vi "Process_All_single.vi"(8 "error in (no error)":errorcluster, 11 "DebuggingTerminal":refnum<class "DebuggingTerminal.lvclass">) -> ()   [LabVIEW 2013, in "MQTT Base.lvlib"]
uses:
  MQTT Base.lvlib
  DebuggingTerminal.lvclass
  Packet Arrival -- cluster.ctl
  <vilib>/LabVIEW Open Source Project/MQTT Control Packets/Control Packets/ControlPacket/ControlPacket.lvclass
  DebuggingTerminal.lvclass/DebuggingTerminal.ctl
  <vilib>/LabVIEW Open Source Project/MQTT Control Packets/Control Packets/ControlPacket/ControlPacket.lvclass/ControlPacket.ctl
  <vilib>/LabVIEW Open Source Project/MQTT Control Packets/Control Packets/MQTT_311/MQTTVersion.lvclass
  <vilib>/LabVIEW Open Source Project/Advanced Structures/Circular Buffers/VariantBuffer/VariantBuffer.lvclass
  PacketFormatter/PacketFormatter.lvclass
panel:
  in  "auto-scroll":bool=TRUE
  out "Incoming":string
  # "MQTT Packets"
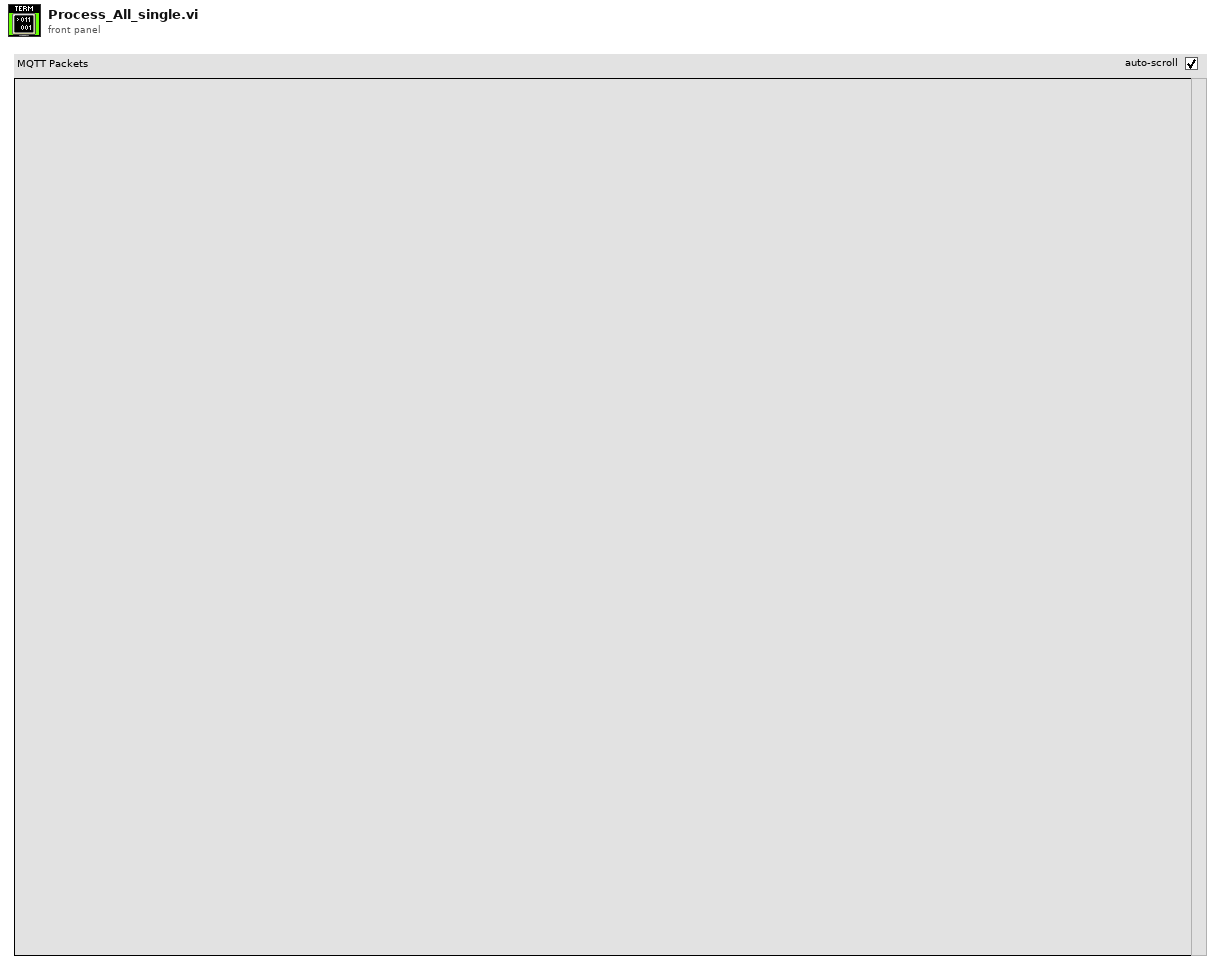
[diagram p1: front panel]
types:
  T1 = typedef "MQTT Base.lvlib/DebuggingTerminal.lvclass/Packet Arrival -- cluster.ctl" = cluster{"Timestamp":timestamp, "Packet":refnum<class "ControlPacket.lvclass">, "Session ID":i32, "outgoing":bool}
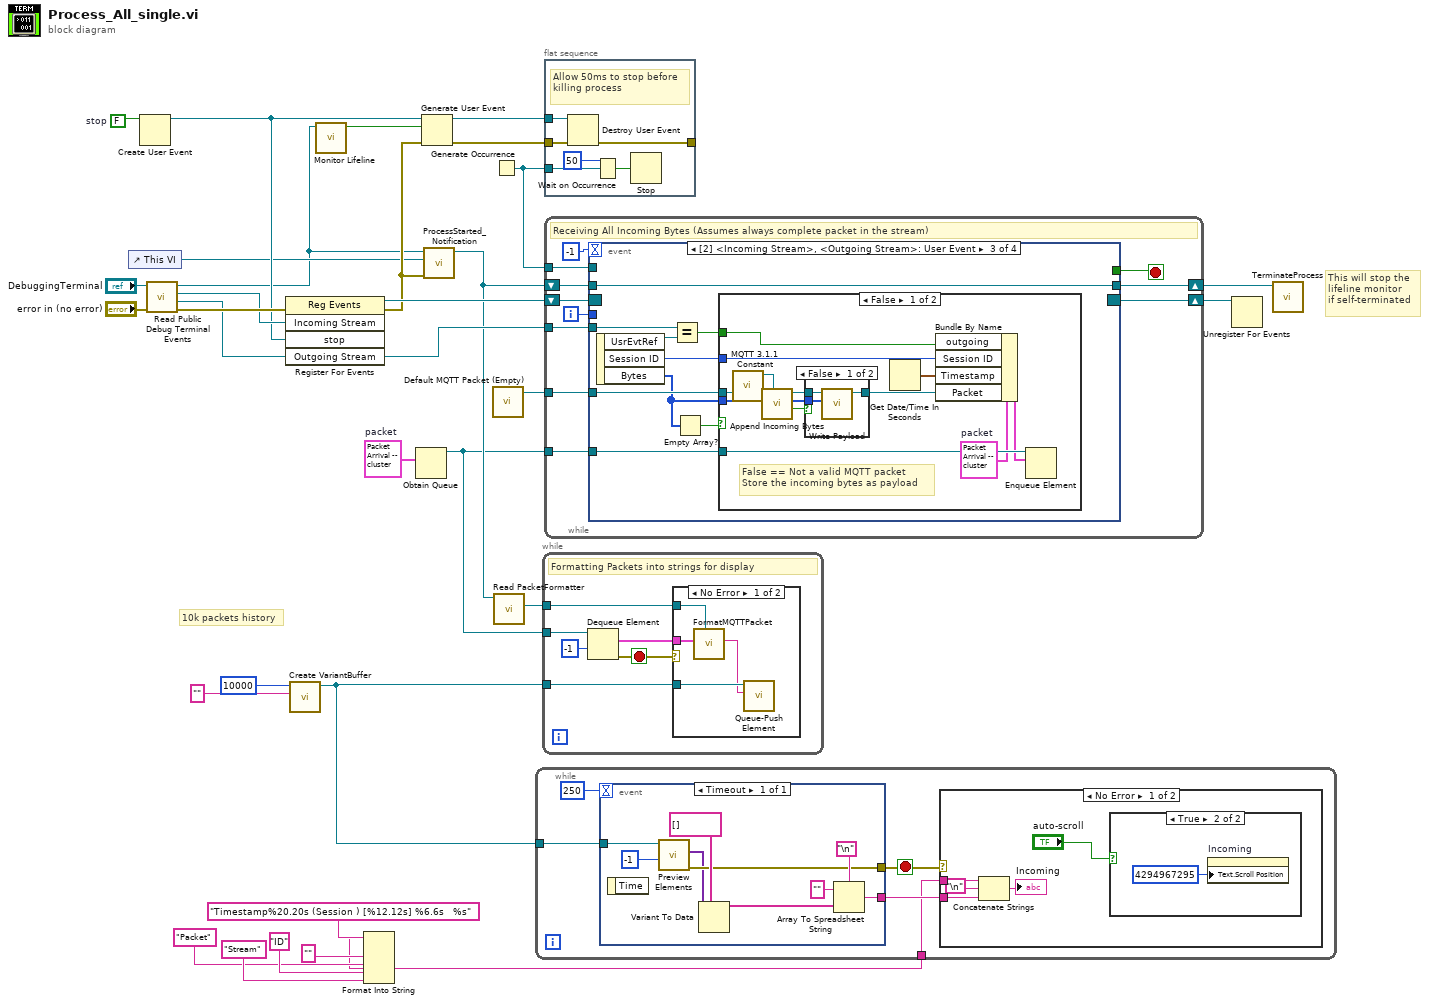
[diagram p0: block diagram]
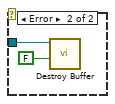
[diagram p2: hidden frame]
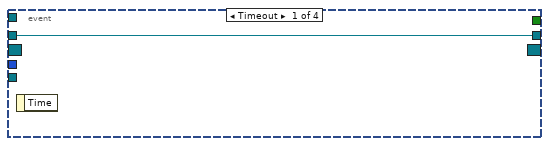
[diagram p5: hidden frame]
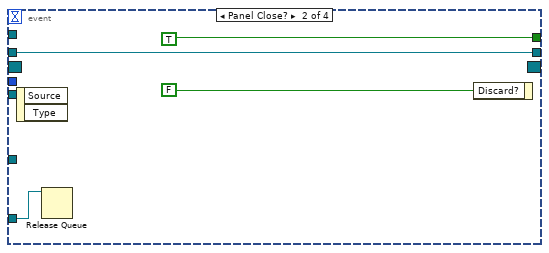
[diagram p6: hidden frame]
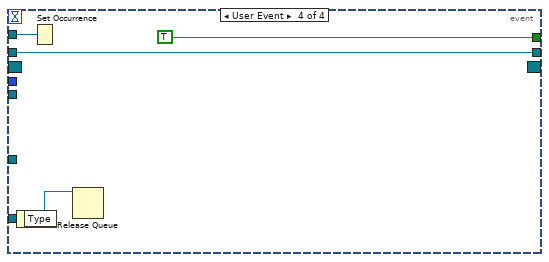
[diagram p9: hidden frame]
diagram:
  w11 = T1 {"Timestamp"=timestamp(0 s since 1904-01-01), "Packet"=refnum, "Session ID"=0, "outgoing"=FALSE}  # packet
  w28 = FALSE  # stop
  # "10k packets history"
  # "This will stop the\nlifeline monitor\nif self-terminated"
  n1 = control-ref of="This VI"() -> (w10:refnum<vi>)
  n2 = Create User Event(user event datatype=w28) -> (user event=w26:refnum<user-event>)  [unwired: 1 in, 1 out]
  n3 = call "Read Public Debug Terminal Events.vi"("error in (no error)"="error in (no error)", "DebuggingTerminal in"="DebuggingTerminal") -> ("error out"=w30:errorcluster, "Outgoing Stream"=w9:refnum<user-event>, "Incoming Stream"=w29:refnum<user-event>, "DebuggingTerminal out"=w6:refnum<class "DebuggingTerminal.lvclass">)  [unwired: 6 in]
  n4 = register-events(error in=w30, w29, w26, w9) -> (reference out=w24:refnum<event-registration>, error out=w18:errorcluster)  [unwired: 1 in]
  n5 = call <vilib>:"Create VariantBuffer.vi"("default"="" ("input 1"), "bufSize"=10000) -> ("Buffer"=w1:refnum<data-value>)  [unwired: 8 in, 1 out]
  n6 = call "Monitor Lifeline.vi"("DebuggingTerminal in"=w6) -> ("Kill Process"=w27:bool)  [unwired: 10 in]
  n7 = Format Into String(format string="Timestamp%20.20s (Session ) [%12.12s] %6.6s   %s", "" ("input 1"), "Packet" ("input 1"), "ID" ("input 1"), "Stream" ("input 1")) -> (resulting string=w5:string)  [unwired: 2 in, 1 out]
  n8 = Obtain Queue(element data type=w11) -> (queue out=w2:refnum<queue>)  [unwired: 4 in, 2 out]
  n9 = Generate User Event(user event=w26, event data cluster=w27, error in=w18) -> (user event out=w25:refnum<user-event>, error out=w19:errorcluster)  [unwired: 1 in]
  n10 = call "ProcessStarted_Notification.vi"("error in (no error)"=w18, "This VI"=w10, "DebuggingTerminal in"=w6) -> ("DebuggingTerminal out"=w3:refnum<class "DebuggingTerminal.lvclass">)  [unwired: 7 in, 1 out]
  n11 = Generate Occurrence() -> (w23:refnum<k4>)
  n12 = call <vilib>:"Default MQTT Packet (Empty).vi"() -> ("No Packet"=w12:refnum<class "ControlPacket.lvclass">)  [unwired: 11 in]
  n13 = call "Read PacketFormatter.vi"("DebuggingTerminal in"=w3) -> ("PacketFormatter"=w4:refnum<class "PacketFormatter.lvclass">)  [unwired: 9 in, 1 out]
  n14 = while {
    tunnel: w5 -> [w34]
    tunnel: w1 -> [w32]
    stop <- w33 stop-if-true
    n15 = event shown="[0] Timeout" {
      selector: _ -> [_]
      dyn-events: _ -> [_]
      timeout: 250 -> [_]
      tunnel: [w46] -> w33
      tunnel: [w47] -> w35
      tunnel: w32 -> [w44]
      event Timeout {
        n16 = event-data() -> ()  [unwired: 1 in, 1 out]
        n17 = call <vilib>:"Preview Elements.vi"("count (-1: all)"=-1, "ByteBuffer in"=w44) -> ("error out"=w46:errorcluster, "elements"=w45:variant[])  [unwired: 7 in, 1 out]
        n18 = Variant To Data(type=string[] [], Variant=w45) -> (data=w50:string[])  [unwired: 1 in, 1 out]
        n19 = Array To Spreadsheet String(delimiter (Tab)="\n", array=w50, 3:"" ("format string")) -> (spreadsheet string=w47:string)
      }
    }
    n20 = case shown="No Error" w33 {
      tunnel: w35 -> [w40 _]
      tunnel: w34 -> [w39 _]
      frame No Error {
        n21 = Concatenate Strings(w39, "\n", w40) -> (→"Incoming":string)
        n22 = case shown="True" "auto-scroll" {
          frame False {
          }
          frame True {
            n23 = property on="Incoming" class="Str"("Text.Scroll Position"=u32 4294967295) -> ()  [unwired: 2 in, 2 out]
          }
        }
      }
      frame Error {
      }
    }
  }
  n24 = while {
    tunnel: w2 -> [w56]
    tunnel: w1 -> [w53]
    tunnel: w4 -> [w52]
    stop <- w57 stop-if-true
    # "Formatting Packets into strings for display"
    n25 = Dequeue Element(queue=w56, timeout in ms (-1)=-1) -> (element=w54:T1, error out=w57:errorcluster)  [unwired: 1 in, 2 out]
    n26 = case shown="No Error" w57 {
      tunnel: w54 -> [w59 _]
      tunnel: w53 -> [w61 w63]
      tunnel: w52 -> [w60 _]
      frame No Error {
        n27 = call "FormatMQTTPacket.vi"("PacketFormatter"=w60, "packet"=w59) -> ("String"=w58:string)  [unwired: 9 in]
        n28 = call <vilib>:"Queue-Push Element.vi"("element"=w58, "Buffer in"=w61) -> ()  [unwired: 5 in, 5 out]
      }
      frame Error {
        n29 = call <vilib>:"Destroy Buffer.vi"("Return Elements (T)"=FALSE, "Buffer"=w63) -> ()  [unwired: 8 in, 2 out]
      }
    }
  }
  n30 = flat-sequence {
    tunnel: w25 -> [w69]
    tunnel: w23 -> [w66]
    tunnel: w19 -> [w65]
    tunnel: [w64] -> _
    frame #0 {
      # "Allow 50ms to stop before killing process"
      n31 = Destroy User Event(user event=w69, error in=w65) -> (error out=w64:errorcluster)
      n32 = Wait on Occurrence(2:w66, 3:50 ("ms timeout (-1)")) -> (0:w67:bool)  [unwired: 1 in]
      n33 = Stop(stop? (T)=w67) -> ()
    }
  }
  n34 = while {
    tunnel: w23 -> [w79]
    shift-right: [w77] -> w22
    shift-left: w24 -> [w80]
    shift-right: [w74] -> w20
    shift-left: w3 -> [w75]
    tunnel: w2 -> [w73]
    tunnel: w12 -> [w72]
    tunnel: w9 -> [w70]
    i -> [w71]
    stop <- w76 stop-if-true
    # "Receiving All Incoming Bytes (Assumes always complete packet in the stream)"
    n35 = event shown="[2] <Incoming Stream>, <Outgoing Stream>: User Event" {
      selector: w80 -> [_ _ _ _]
      dyn-events: [_ _ _ _] -> w77
      timeout: -1 -> [_ _ _ _]
      tunnel: w79 -> [_ _ _ w115]
      tunnel: [_ TRUE ("Discard?") _ TRUE] -> w76
      tunnel: w75 -> [w81 w85 w94 w113]
      tunnel: [w81 w85 w94 w113] -> w74
      tunnel: w73 -> [_ w82 w93 w112]
      tunnel: w72 -> [_ _ w91 _]
      tunnel: w71 -> [_ _ _ _]
      tunnel: w70 -> [_ _ w87 _]
      event Timeout {
        n36 = event-data() -> ()  [unwired: 1 in, 1 out]
      }
      event Panel Close? {
        n37 = event-data() -> ()  [unwired: 1 in, 2 out]
        n38 = Release Queue(queue=w82) -> ()  [unwired: 2 in, 3 out]
        n39 = event-data("Discard?"=FALSE) -> ()  [unwired: 1 in, 1 out]
      }
      event User Event {
        n40 = event-data() -> ("UsrEvtRef"=w88:refnum<user-event>, "Session ID"=w92:i32, "Bytes"=w90:u8[])  [unwired: 1 in]
        n41 = Equal?(x=w87, y=w88) -> (x = y?=w86:bool)
        n42 = Empty Array?(array=w90) -> (empty?=w89:bool)
        n43 = case shown="False" w89 {
          tunnel: w93 -> [w106 _]
          tunnel: w92 -> [w105 _]
          tunnel: w91 -> [w104 _]
          tunnel: w90 -> [w96 _]
          tunnel: w86 -> [w95 _]
          frame False {
            w101 = T1 {"Timestamp"=timestamp(0 s since 1904-01-01), "Packet"=refnum, "Session ID"=0, "outgoing"=FALSE}  # packet
            # "False == Not a valid MQTT packet\nStore the incoming bytes as payload"
            n44 = call <vilib>:"MQTT 3.1.1 Constant.vi"() -> ("MQTT 3.1.1"=w107:refnum<class "MQTTVersion.lvclass">)  [unwired: 11 in]
            n45 = call <vilib>:"Append Incoming Bytes.vi"("MQTT Version (3.1.1)"=w107, "Incoming Packets"=w96, "Incomplete ControlPacket"=w104) -> ("Complete Packet"=w100:bool, "Remaining Packets"=w97:u8[], "ControlPacket"=w98:refnum<class "ControlPacket.lvclass">)  [unwired: 5 in, 1 out]
            n46 = case shown="False" w100 {
              tunnel: [w109 w111] -> w99
              tunnel: w98 -> [w110 w111]
              tunnel: w97 -> [w108 _]
              frame False {
                n47 = call <vilib>:"Write Payload.vi"("Payload"=w108, "ControlPacket in"=w110) -> ("ControlPacket out"=w109:refnum<class "ControlPacket.lvclass">)  [unwired: 9 in]
              }
              frame True {
              }
            }
            n48 = Get Date/Time In Seconds() -> (seconds since 1Jan1904=w102:timestamp)
            n49 = Bundle By Name(cluster=w101, "outgoing"=w95, "Session ID"=w105, "Timestamp"=w102, "Packet"=w99) -> (w103:T1)
            n50 = Enqueue Element(queue=w106, element=w103) -> ()  [unwired: 2 in, 3 out]
          }
          frame True {
          }
        }
      }
      event User Event {
        n51 = event-data() -> ()  [unwired: 1 in, 1 out]
        n52 = Set Occurrence(w115) -> ()
        n53 = Release Queue(queue=w112) -> ()  [unwired: 2 in, 3 out]
      }
    }
  }
  n54 = Unregister For Events(event registration refnum=w22) -> ()  [unwired: 1 in, 1 out]
  n55 = call "TerminateProcess.vi"("DebuggingTerminal in"=w20) -> ()  [unwired: 10 in, 1 out]
